vi "User_Change_Password.vi"(11 "User_Name":string caption="用  户  名") -> ()   [LabVIEW 2020]
panel:
  in  "Confirm Password":string caption="确认密码"
  in  "New Password":string caption="新  密  码"
  in  "Last Password":string caption="旧  密  码"
  in  "Ok":bool
  # "修改密码"
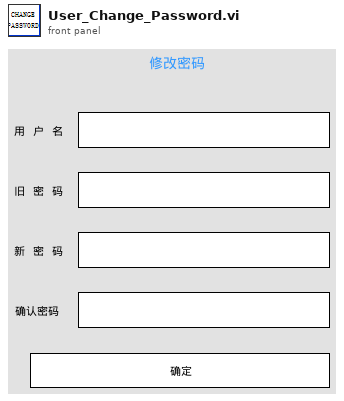
[diagram p1: front panel]
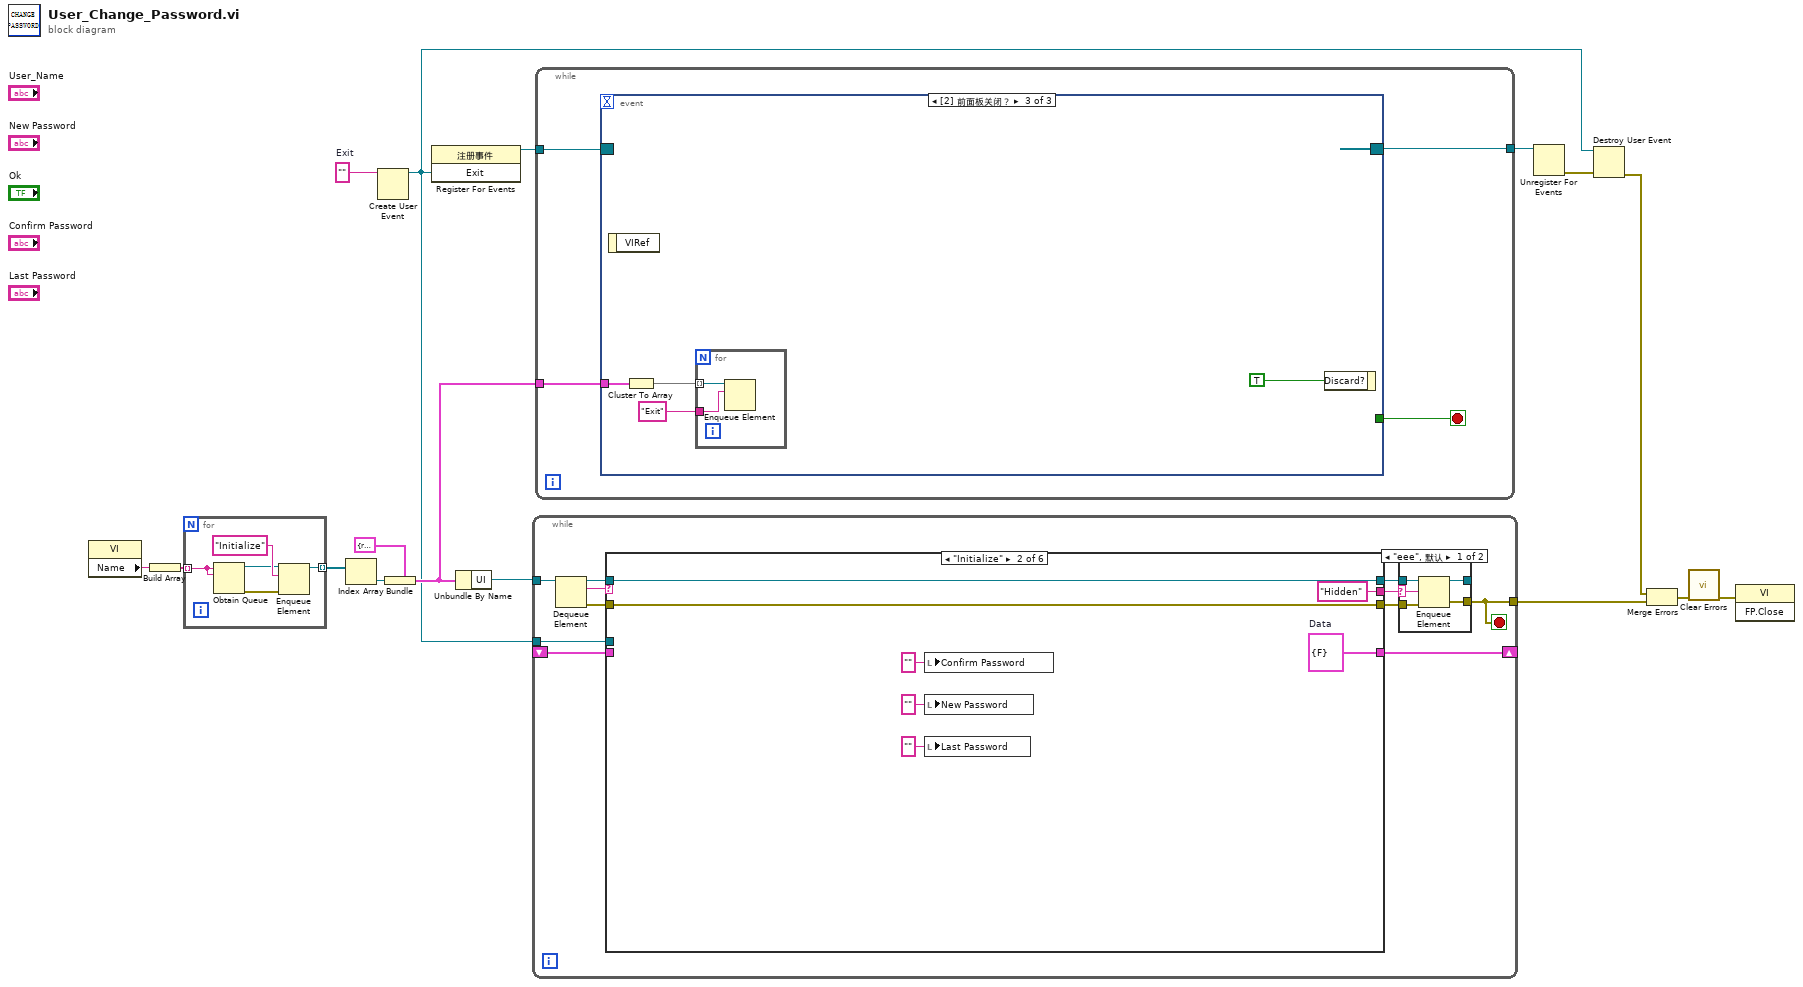
[diagram p0: block diagram]
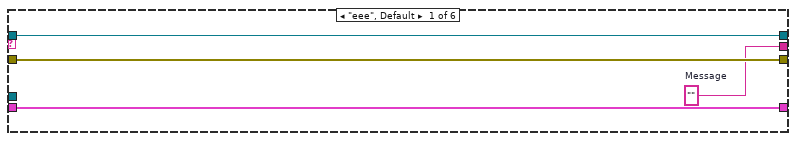
[diagram p3: hidden frame]
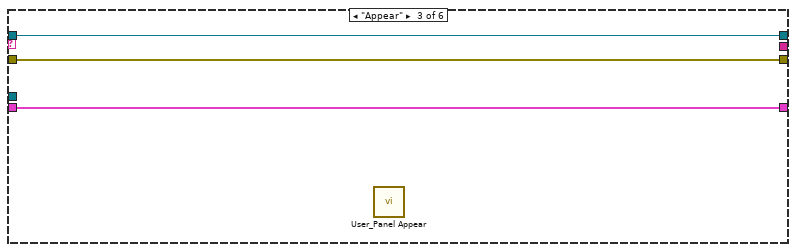
[diagram p4: hidden frame]
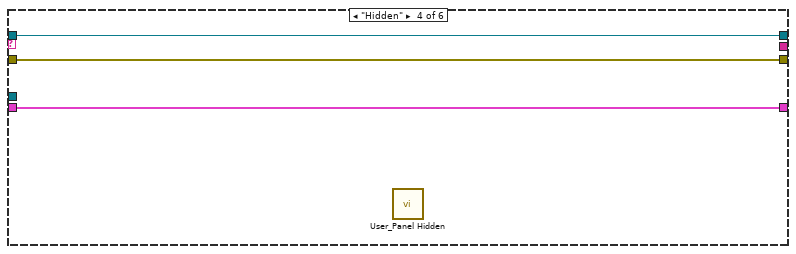
[diagram p5: hidden frame]
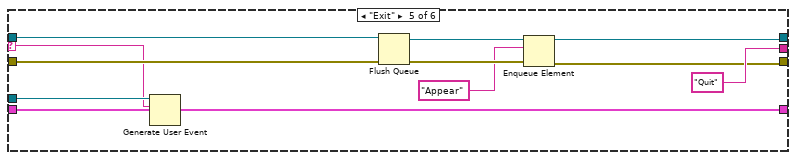
[diagram p6: hidden frame]
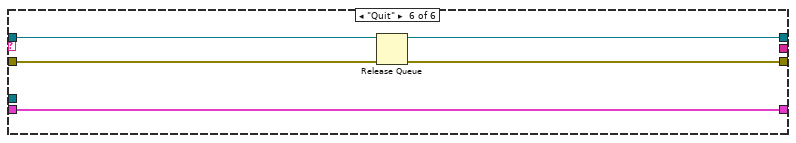
[diagram p7: hidden frame]
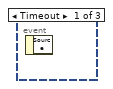
[diagram p8: hidden frame]
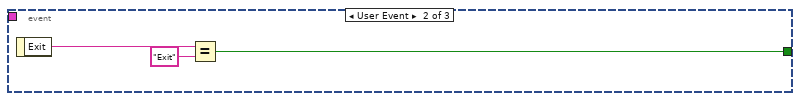
[diagram p9: hidden frame]
diagram:
  w2 = ""  # Exit
  n1 = property class="VI"() -> ("Name"=w12:string)  [unwired: 2 in, 2 out]
  n2 = Build Array(w12) -> (w13:string[])
  n3 = for {
    tunnel: w13 -> [w17] mode=indexing
    tunnel: [w18] -> w7 mode=indexing
    n4 = Obtain Queue(name (unnamed)=w17, element data type=w17) -> (queue out=w20:refnum<queue>, error out=w19:errorcluster)  [unwired: 3 in, 1 out]
    n5 = Enqueue Element(queue=w20, element="Initialize" ("元素"), error in (no error)=w19) -> (queue out=w18:refnum<queue>)  [unwired: 1 in, 2 out]
  }
  n6 = Index Array(array=w7) -> (element=w10:refnum<queue>)  [unwired: 1 in]
  n7 = Create User Event(user event datatype=w2) -> (user event=w6:refnum<user-event>)  [unwired: 1 in, 1 out]
  n8 = Bundle(cluster=cluster{"UI":refnum<queue>} {"UI"=refnum}, "UI"=w10) -> (w11:cluster{"UI":refnum<queue>})
  n9 = register-events(w6) -> (reference out=w3:refnum<event-registration>)  [unwired: 2 in, 1 out]
  n10 = Unbundle By Name(w11) -> ("UI"=w8:refnum<queue>)
  n11 = while {
    tunnel: w8 -> [w32]
    tunnel: [w22] -> w15
    shift-right: [w26] -> _
    shift-left: _ -> [w25]
    tunnel: w6 -> [w24]
    stop <- w22 stop-if-true
    n12 = Dequeue Element(queue=w32) -> (queue out=w31:refnum<queue>, element=w23:string, error out=w28:errorcluster)  [unwired: 2 in, 1 out]
    n13 = case shown="\"Initialize\"" w23 {
      selector: w23 -> [_ _ _ _ w62 _]
      tunnel: w31 -> [w43 w50 w53 w56 w65 w71]
      tunnel: [w43 w50 w53 w56 w60 w71] -> w30
      tunnel: [w42 w49 w52 w55 w58 w68] -> w29
      tunnel: w28 -> [w42 w49 w52 w55 w64 w70]
      tunnel: [w41 "Hidden" ("Message") _ _ "Quit" ("Message") _] -> w27
      tunnel: [w40 w48 w51 w54 w67 w69] -> w26
      tunnel: w25 -> [w40 _ w51 w54 w67 w69]
      tunnel: w24 -> [_ _ _ _ w63 _]
      frame "eee", Default {
        w41 = ""  # Message
      }
      frame "Initialize" {
        w48 = cluster{"Data":bool} {"Data"=FALSE}  # Data
        n14 = local write "Confirm Password"("" ("Confirm Password")) -> ()
        n15 = local write "New Password"("" ("New Password")) -> ()
        n16 = local write "Last Password"("" ("Last Password")) -> ()
      }
      frame "Appear" {
        n17 = call "User_Panel Appear.vi"() -> ()  [unwired: 11 in, 1 out]
      }
      frame "Hidden" {
        n18 = call "User_Panel Hidden.vi"() -> ()  [unwired: 11 in, 1 out]
      }
      frame "Exit" {
        n19 = Generate User Event(user event=w63, event data cluster=w62) -> ()  [unwired: 2 in, 2 out]
        n20 = Flush Queue(queue=w65, error in (no error)=w64) -> (queue out=w61:refnum<queue>, error out=w59:errorcluster)  [unwired: 1 out]
        n21 = Enqueue Element(queue=w61, element="Appear" ("元素"), error in (no error)=w59) -> (queue out=w60:refnum<queue>, error out=w58:errorcluster)  [unwired: 1 in, 1 out]
      }
      frame "Quit" {
        n22 = Release Queue(queue=w71, error in (no error)=w70) -> (error out=w68:errorcluster)  [unwired: 1 in, 2 out]
      }
    }
    n23 = case shown="\"eee\", 默认" w27 {
      selector: w27 -> [w33 _]
      tunnel: w30 -> [w37 w39]
      tunnel: w29 -> [w36 w38]
      tunnel: [w35 w38] -> w22
      tunnel: [w34 w39] -> _
      frame "eee", Default {
        n24 = Enqueue Element(queue=w37, element=w33, error in (no error)=w36) -> (queue out=w34:refnum<queue>, error out=w35:errorcluster)  [unwired: 1 in, 1 out]
      }
      frame "" {
      }
    }
  }
  n25 = while {
    tunnel: w3 -> [w74]
    tunnel: [w73] -> w5
    tunnel: w11 -> [w72]
    stop <- w75 stop-if-true
    n26 = event shown="[2] 前面板关闭？" {
      selector: w74 -> [_ _ _]
      dyn-events: [_ _ _] -> w73
      timeout: _ -> [_ _ _]
      tunnel: [_ w77 _] -> w75
      tunnel: w72 -> [_ _ w81]
      event Timeout {
        n27 = event-data() -> ()  [unwired: 1 in, 1 out]
      }
      event User Event {
        n28 = event-data() -> ("Exit"=w78:string)  [unwired: 1 in]
        n29 = Equal?(x=w78, y="Exit") -> (x = y?=w77:bool)
      }
      event Panel Close? {
        n30 = event-data() -> ()  [unwired: 1 in, 1 out]
        n31 = Cluster To Array(cluster=w81) -> (array=w80:refnum<queue>[])
        n32 = for {
          tunnel: w80 -> [w84] mode=indexing
          tunnel: "Exit" ("元素") -> [w83]
          n33 = Enqueue Element(queue=w84, element=w83) -> ()  [unwired: 2 in, 3 out]
        }
        n34 = event-data("Discard?"=TRUE ("放弃？")) -> ()  [unwired: 1 in, 1 out]
      }
    }
  }
  n35 = Unregister For Events(event registration refnum=w5) -> (error out=w4:errorcluster)  [unwired: 1 in]
  n36 = Destroy User Event(user event=w6, error in=w4) -> (error out=w14:errorcluster)
  n37 = Merge Errors(w14, w15) -> (w16:errorcluster)
  n38 = call <vilib>:"Clear Errors.vi"("error in (no error)"=w16) -> ("error out"=w1:errorcluster)  [unwired: 5 in, 1 out]
  n39 = invoke class="VI" method="FP.Close"(error in=w1) -> ()  [unwired: 2 in, 3 out]
